vi "Emballage_fichierSpecifique.vi"(8 "error in (no error)":errorcluster caption="entrée d'erreur (pas d'erreur)", 10 "Tableau n° valves":string[](array[string]), 11 "ID_ARTICLE":string) -> (0 "error out":errorcluster caption="sortie d'erreur")   [LabVIEW 2020]
uses:
  Modules/FS/60_FS_Controles/60_FS_SetGet.ctl
  <vilib>/Utility/NIReport.llb/Report Type.ctl
  <vilib>/drjdpowell/SQLite Library/SQL Connection/Open (path).vi
  <vilib>/drjdpowell/SQLite Library/SQL Connection/Open (string).vi
  <vilib>/AdvancedString/Path To Command Line String.vi
  <vilib>/Utility/NIReport.llb/Append Text Table to Report (wrap).vi
  <vilib>/drjdpowell/SQLite Library/SQL Connection/Connection.lvclass
  <vilib>/Utility/NIReport.llb/NI_report.lvclass
  <vilib>/Utility/NIReport.llb/NI_ReportGenerationCore.lvlib
  <vilib>/Utility/NIReport.llb/Excel/NI_Excel.lvclass
panel:
  out "chaîne résultante":string
  out "Number of Files":i32 caption="Nombre de fichiers"
  out "All Files in Dir":path[](array[path]) caption="Tous les fichiers du rép."
  out "Result Set":string[][](table) caption="Result Set (from first statement with results)"
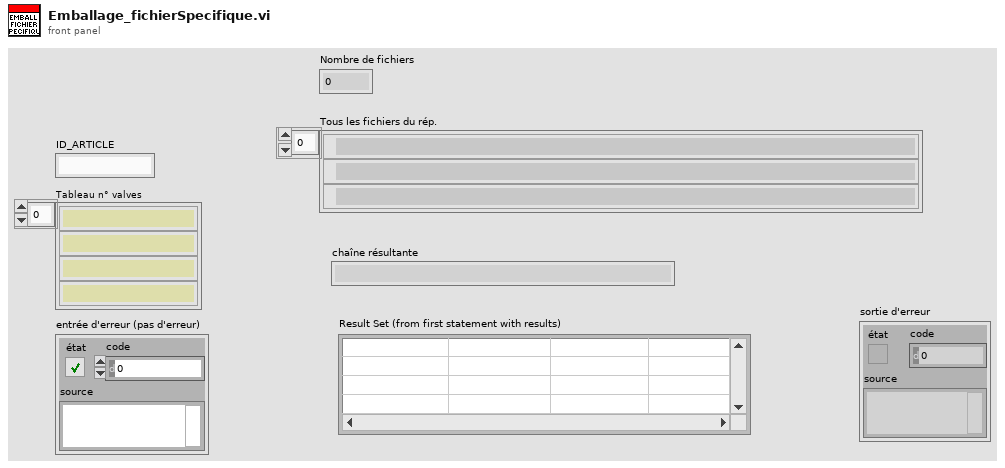
[diagram p1: front panel]
types:
  T1 = typedef "60_FS_SetGet.ctl" = enum16{"set", "get"}
  T2 = cluster{"position (Excel)":cluster{"row":i32, "column":i32}, "name (Excel)":string, "bookmark (Word)":string}
  T3 = typedef "NI_ReportGenerationCore.lvlib/Report Type.ctl" = enum16{"HTML", "Word", "Excel"}
  T4 = typedef "60_FS_CLT_Chemins.ctl" = cluster{"Racine_local":path, "Racine_reseau":path, "Racine_Support_Application":path, "Fichier_Journalisation":path, "Connexion_BDD_VSX":path, "Connexion_BDD_PLZ":path}
  T5 = cluster{"on/off":bool, "weight":i32, "color":u32}
  T6 = cluster{"start (wd) - row (xl) ":i32, "end (wd) - col (xl) ":i32}
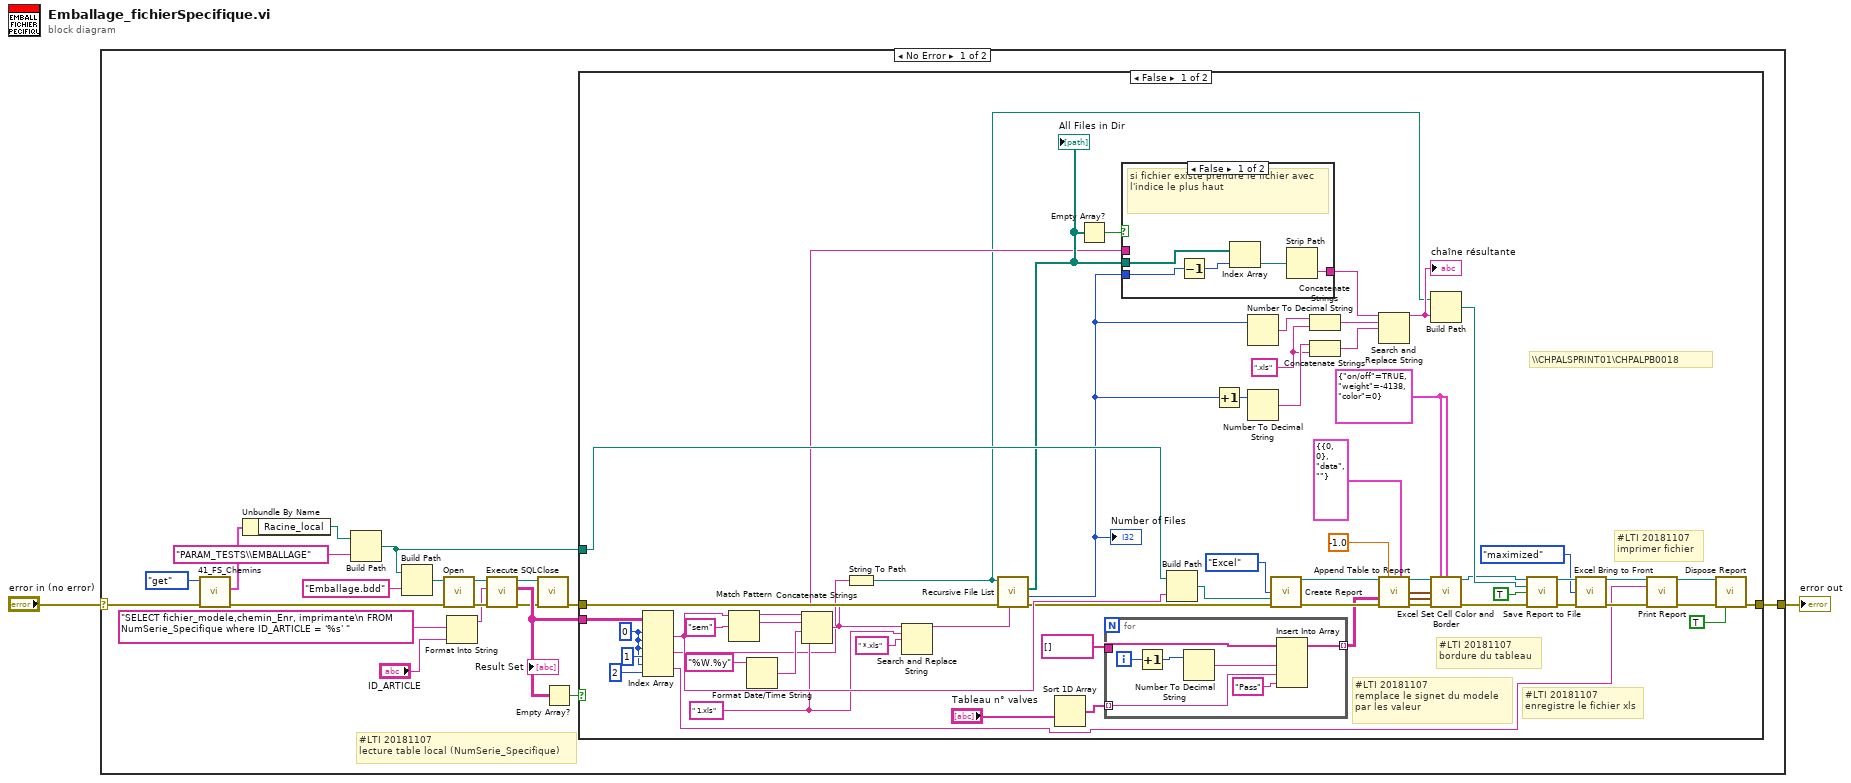
[diagram p0: block diagram]
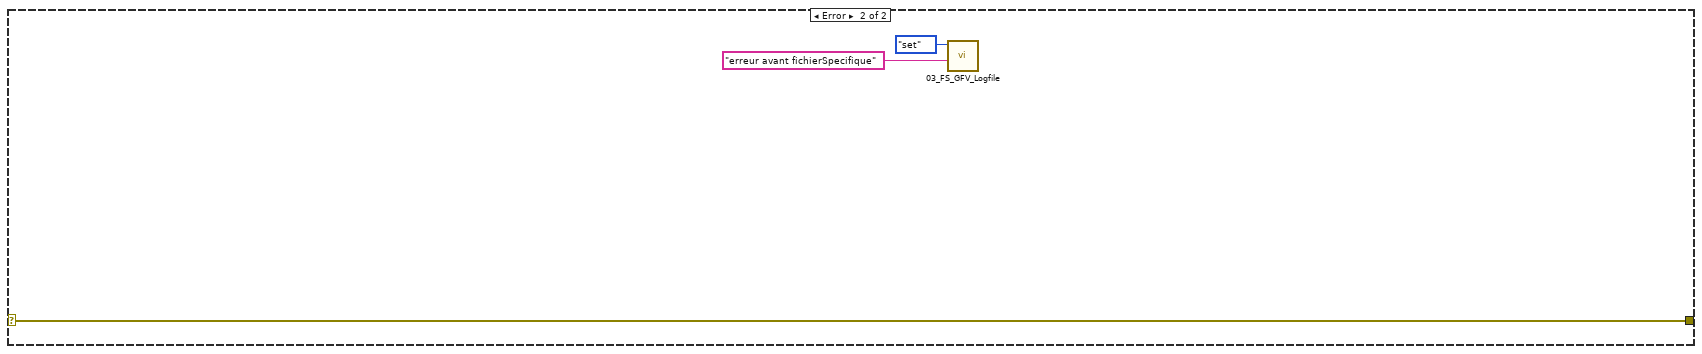
[diagram p4: hidden frame]
diagram:
  n1 = case shown="No Error" "error in (no error)" {
    selector: "error in (no error)" -> [w4 w96]
    tunnel: [w3 w96] -> w1
    frame No Error {
      # "#LTI 20181107\nlecture table local (NumSerie_Specifique)"
      n2 = call "41_FS_Chemins.vi"("error in (no error)"=w4, "SetGet"=60_FS_SetGet."get") -> ("error out"=w20:errorcluster, "CLT_Chemins_out"=w9:T4)  [unwired: 8 in]
      n3 = Unbundle By Name(w9) -> ("Racine_local"=w11:path)
      n4 = Build Path(base path=w11, name or relative path="PARAM_TESTS\\EMBALLAGE" ("nom ou chemin relatif")) -> (appended path=w13:path)
      n5 = Build Path(base path=w13, name or relative path="Emballage.bdd" ("nom ou chemin relatif")) -> (appended path=w22:path)
      n6 = call-poly <vilib>:"Open.vi"("error in (no error)"=w20, "db file"=w22) -> ("error out"=w19:errorcluster, "SQLite Connection"=w21:refnum<class "Connection.lvclass">)  [unwired: 8 in]
      n7 = Format Into String(format string="SELECT fichier_modele,chemin_Enr, imprimante\n FROM NumSerie_Specifique where ID_ARTICLE = '%s' " ("SQL"), "ID_ARTICLE") -> (resulting string=w17:string)  [unwired: 2 in, 1 out]
      n8 = call <vilib>:"Execute SQL.vi"("error in (no error)"=w19, "SQL"=w17, "SQLite Connection in"=w21) -> ("error out"=w5:errorcluster, "Result Set"=w14:string[][], "SQLite Connection"=w6:refnum<class "Connection.lvclass">)  [unwired: 5 in, 1 out]
      "Result Set" <- w14
      n9 = call-dynamic "Close.vi"("error in (no error)"=w5, "SQLite Connection in"=w6) -> ("error out"=w7:errorcluster)  [unwired: 9 in]
      n10 = Empty Array?(array=w14) -> (empty?=w15:bool)
      n11 = case shown="False" w15 {
        tunnel: w14 -> [w72 _]
        tunnel: w13 -> [w71 _]
        tunnel: w7 -> [w61 w95]
        tunnel: [w44 w95] -> w3
        frame False {
          w33 = T5 {"on/off"=TRUE, "weight"=-4138, "color"=0} ("outside border")
          w53 = ".xls" ("chaîne")
          w59 = " 1.xls" ("chaîne")
          w27 = 0 ("indice (ligne)")
          # "#LTI 20181107\nimprimer fichier"
          # "\\\\CHPALSPRINT01\\CHPALPB0018"
          # "#LTI 20181107\nbordure du tableau"
          # "#LTI 20181107\nenregistre le fichier xls"
          # "#LTI 20181107\nremplace le signet du modele\npar les valeur"
          n12 = Index Array(array=w72, index (row) #1=w27, index (col) #1=w27, index (row) #2=w27, index (col) #2=1 ("indice désactivé (col)"), index (row) #3=w27, index (col) #3=2 ("indice désactivé (col)")) -> (element #1=w69:string, element #2=w24:string, element #3=w25:string)
          n13 = Match Pattern(string=w69, regular expression="sem" ("expression régulière")) -> (before substring=w68:string, match substring=w66:string)  [unwired: 1 in, 2 out]
          n14 = Format Date/Time String(time format string (%c)="%W.%y" ("chaîne de format de l'heure (%c)")) -> (date/time string=w64:string)  [unwired: 2 in]
          n15 = Concatenate Strings(w68, w66, w64, w59) -> (w45:string)
          n16 = String To Path(string=w24) -> (path=w23:path)
          n17 = Search and Replace String(input string=w45, search string=w59, replace string=" *.xls" ("chaîne de remplacement (\"\")")) -> (result string=w46:string)  [unwired: 5 in, 3 out]
          n18 = call <vilib>:"Recursive File List.vi"("pattern"=w46, "error in (no error)"=w61, "Folder Path"=w23) -> ("error out"=w60:errorcluster, "Number of Files"=w50:i32, "All Files in Dir"=w48:path[])  [unwired: 4 in, 2 out]
          "Number of Files" <- w50
          "All Files in Dir" <- w48
          n19 = Sort 1D Array(array="Tableau n° valves") -> (sorted array=w40:string[])
          n20 = Empty Array?(array=w48) -> (empty?=w49:bool)
          n21 = for {
            tunnel: w40 -> [w84] mode=indexing
            tunnel: string[] [] -> [w88]
            tunnel: [w82] -> w41 mode=indexing
            i -> [w87]
            n22 = Increment(x=w87) -> (x+1=w86:i32)
            n23 = Number To Decimal String(number=w86) -> (decimal integer string=w85:string)  [unwired: 1 in]
            n24 = Insert Into Array(array=w88, new element #1=w85, new element #2=w84, new element #3="Pass" ("nouvel élément/sous-tableau")) -> (w82:string[])  [unwired: 1 in]
          }
          n25 = case shown="False" w49 {
            tunnel: w48 -> [w93 _]
            tunnel: w50 -> [w91 _]
            tunnel: [w89 w94] -> w47
            tunnel: w45 -> [_ w94]
            frame False {
              # "si fichier existe prendre le fichier avec l'indice le plus haut"
              n26 = Decrement(x=w91) -> (x-1=w92:i32)
              n27 = Index Array(array=w93, index=w92) -> (element=w90:path)
              n28 = Strip Path(path=w90) -> (name=w89:string)  [unwired: 1 out]
            }
            frame True {
              # "le fichier n'existe pas"
            }
          }
          n29 = Build Path(base path=w71, name or relative path=w69) -> (appended path=w70:path)
          n30 = Increment(x=w50) -> (x+1=w57:i32)
          n31 = Number To Decimal String(number=w50) -> (decimal integer string=w56:string)  [unwired: 1 in]
          n32 = Number To Decimal String(number=w57) -> (decimal integer string=w58:string)  [unwired: 1 in]
          n33 = call <vilib>:"Create Report.vi"("report type"=Report_Type."Excel" ("Report Type"), "template (empty)"=w70, "error in (no error)"=w60) -> ("report out"=w78:refnum<class "NI_report.lvclass">, "error out"=w79:errorcluster)  [unwired: 11 in]
          n34 = Concatenate Strings(w56, w53) -> (w55:string)
          n35 = Concatenate Strings(w58, w53) -> (w54:string)
          n36 = Search and Replace String(input string=w47, search string=w55, replace string=w54) -> (result string=w52:string)  [unwired: 5 in, 3 out]
          "chaîne résultante" <- w52
          n37 = call-poly <vilib>:"Append Table to Report.vi"("report in"=w78, "column width (1)"=-1.0, "MS Office parameters"=T2 {"position (Excel)"={"row"=0, "column"=0}, "name (Excel)"="data", "bookmark (Word)"=""}, "text data"=w41, "error in (no error)"=w79) -> ("report out"=w37:refnum<class "NI_report.lvclass">, "range (wd) - start (xl)"=w39:T6, "end (xl)"=w38:cluster{"row (xl) ":i32, "col (xl) ":i32}, "error out"=w35:errorcluster)  [unwired: 7 in]
          n38 = Build Path(base path=w23, name or relative path=w52) -> (appended path=w51:path)
          n39 = call <vilib>:"Excel Set Cell Color and Border.vi"("report in"=w37, "inside border"=w33, "outside border"=w33, "start (-1, -1)"=w39, "end (-1, -1)"=w38, "error in (no error)"=w35) -> ("report out"=w36:refnum<class "NI_report.lvclass">, "error out"=w34:errorcluster)  [unwired: 8 in]
          n40 = call-dynamic "Save Report to File.vi"("report in"=w36, "report file path"=w51, "prompt to replace? (F)"=TRUE, "error in (no error)"=w34) -> ("report out"=w80:refnum<class "NI_report.lvclass">, "error out"=w81:errorcluster)  [unwired: 10 in]
          n41 = call <vilib>:"Excel Bring to Front.vi"("report in"=w80, "window state (maximized)"=enum16{"maximized", "minimized", "normal"}."maximized", "error in (no error)"=w81) -> ("report out"=w29:refnum<class "NI_report.lvclass">, "error out"=w32:errorcluster)  [unwired: 11 in]
          n42 = call-dynamic "Print Report.vi"("report in"=w29, "printer name (default)"=w25, "error in (no error)"=w32) -> ("report out"=w30:refnum<class "NI_report.lvclass">, "error out"=w31:errorcluster)  [unwired: 11 in]
          n43 = call-dynamic "Dispose Report.vi"("report in"=w30, "error in (no error)"=w31, "close report? (T)"=TRUE) -> ("error out"=w44:errorcluster)  [unwired: 12 in]
        }
        frame True {
          # "tableau vide donc pas de fichier spécifique pour le produit sélectionné"
        }
      }
    }
    frame Error {
      n44 = call "03_FS_GFV_Logfile.vi"("Chaîne"="erreur avant fichierSpecifique", "States"=60_FS_SetGet."set") -> ()  [unwired: 8 in, 2 out]
    }
  }
  "error out" <- w1
